vi "Display Global VI.vi"() -> ()   [LabVIEW 2012]
panel:
  in  "Card #":dbl
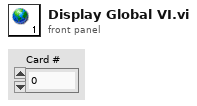
[diagram p1: front panel]
diagram:
